vi "数据查询_仪器数据.vi"() -> ()   [LabVIEW 2016]
uses:
  <vilib>/Utility/miscctls.llb/LVRowAndColumnUnsignedTypeDef.ctl
  <vilib>/Utility/miscctls.llb/LVPointTypeDef.ctl
  <userlib>/_OpenG.lib/array/array.llb/Sort 2D Array (String)__ogtk.vi
  <userlib>/_OpenG.lib/array/array.llb/Sort 1D Array (I32)__ogtk.vi
panel:
  in  "下拉列表":string(xcontrol)
  in  "导出":bool
  out "数据筛选_分钟小时":string(combo)="实时数据"
  out "数据筛选_工作类型":string(combo)="全部数据"
  in  "查询":bool
  in  "结束日期":string="2050/01/01"
  in  "起始日期":string="2010/01/01"
  in  "数据表":T1
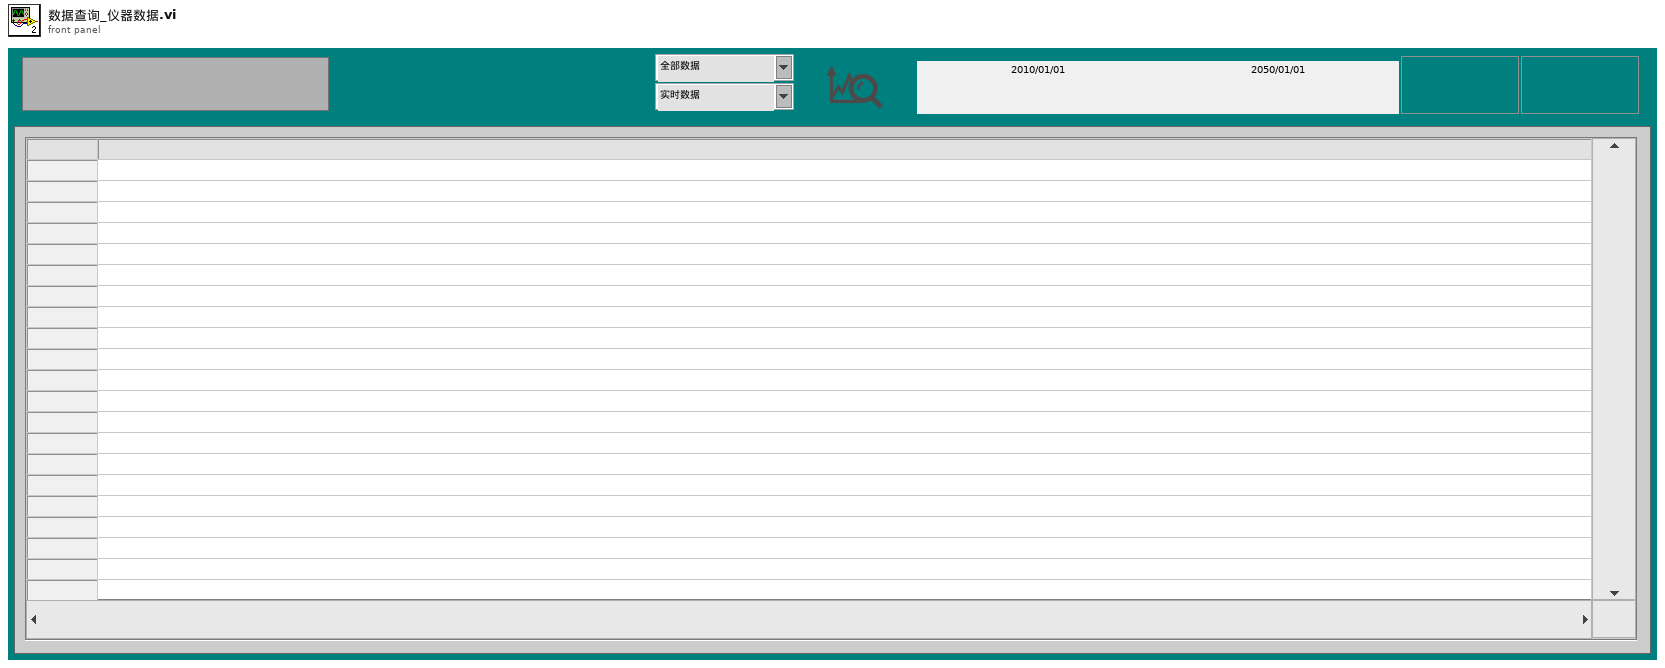
[diagram p1: front panel]
types:
  T1 = typedef "数据查询大列表框.ctl" = i32
  T2 = enum16{"Not Moving", "Mouse Down", "Douse Up", "Moving"}
  T3 = typedef "LVRowAndColumnUnsignedTypeDef.ctl" = cluster{"Row":u32, "Column":u32}
  T4 = typedef "LVPointTypeDef.ctl" = cluster{"Horizontal":i16, "Vertical":i16}
  T5 = cluster{"时间标识":timestamp, "设备":string, "日志信息":string, "流程参数":string}
  T6 = typedef "LVPoint32TypeDef.ctl" = cluster{"Horizontal":i32, "Vertical":i32}
  T7 = typedef "LVRowAndColumnTypeDef.ctl" = cluster{"Row":i32, "Column":i32}
  T8 = enum8{"Enabled", "Disabled", "Disabled and Grayed Out"}
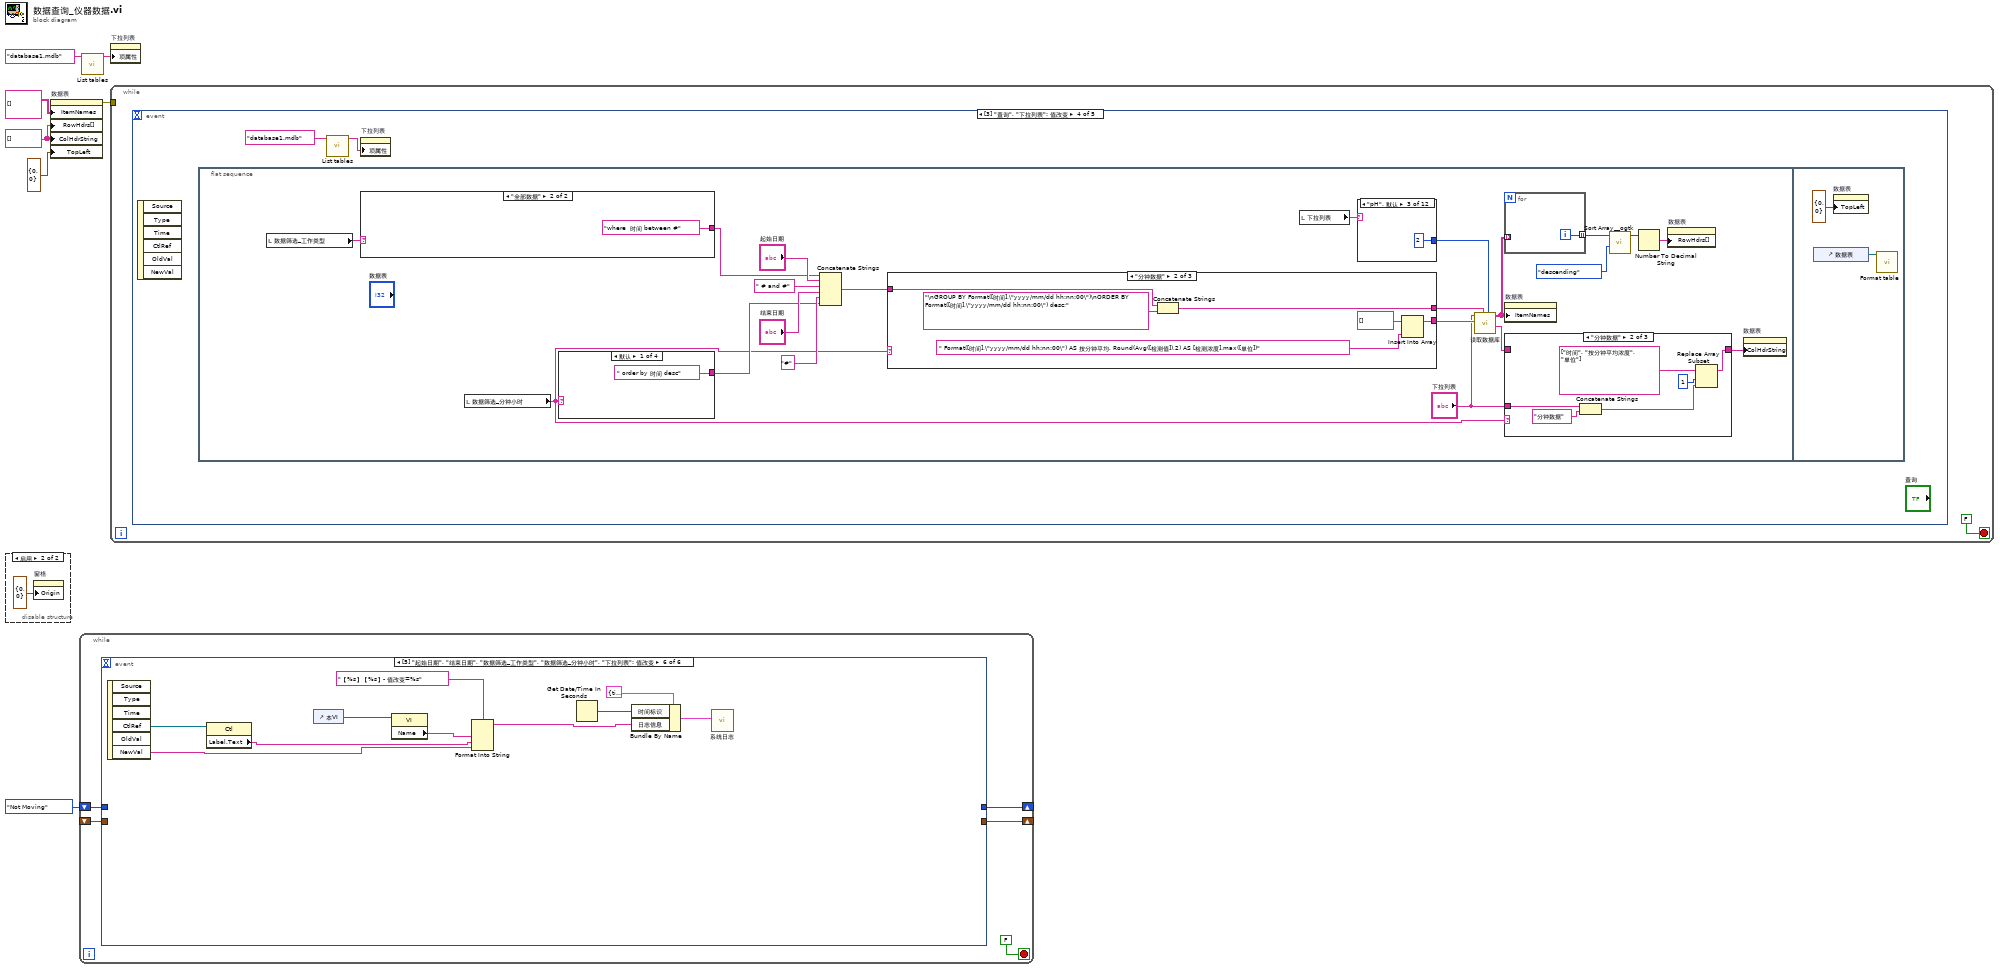
[diagram p0: block diagram]
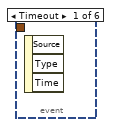
[diagram p2: hidden frame]
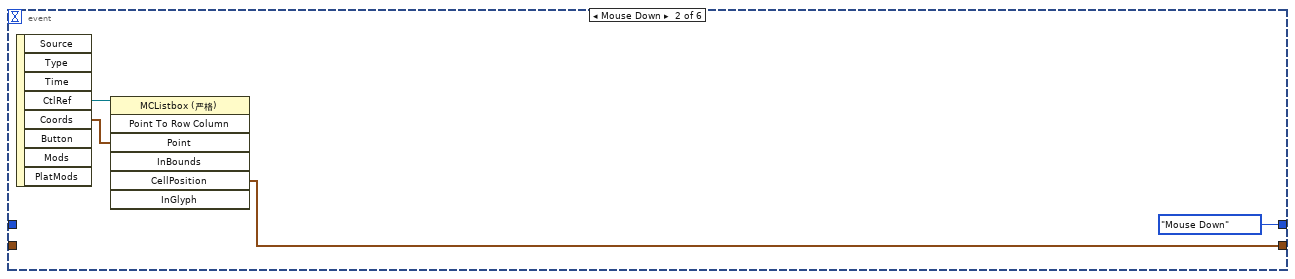
[diagram p3: hidden frame]
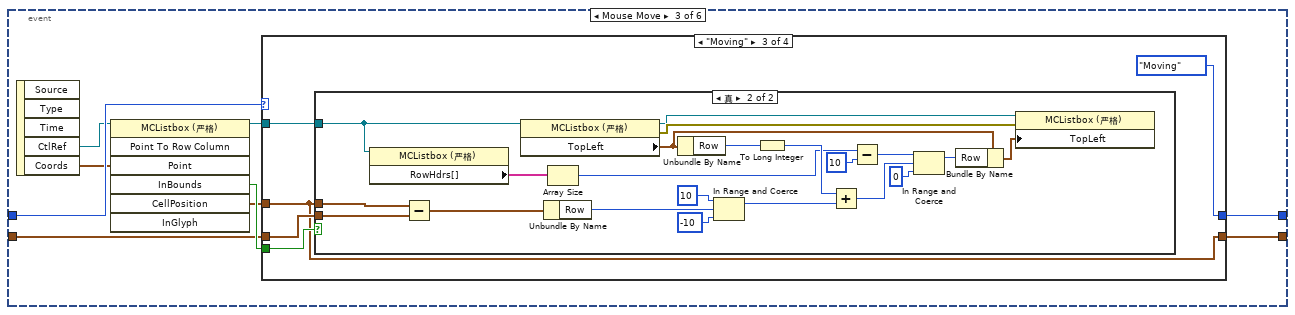
[diagram p4: hidden frame]
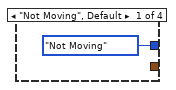
[diagram p5: hidden frame]
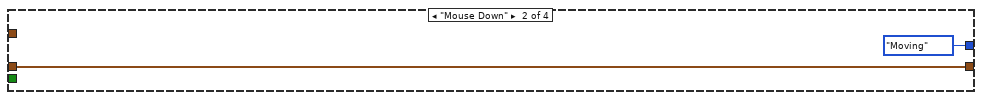
[diagram p6: hidden frame]
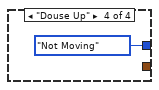
[diagram p8: hidden frame]
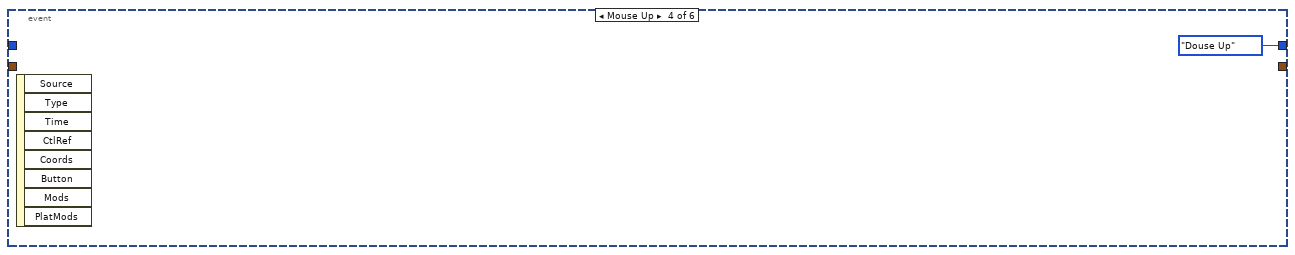
[diagram p9: hidden frame]
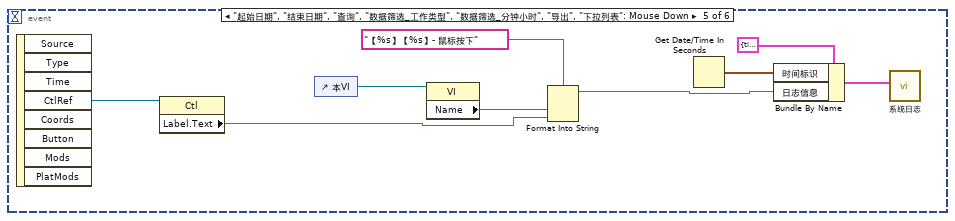
[diagram p10: hidden frame]
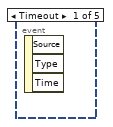
[diagram p11: hidden frame]
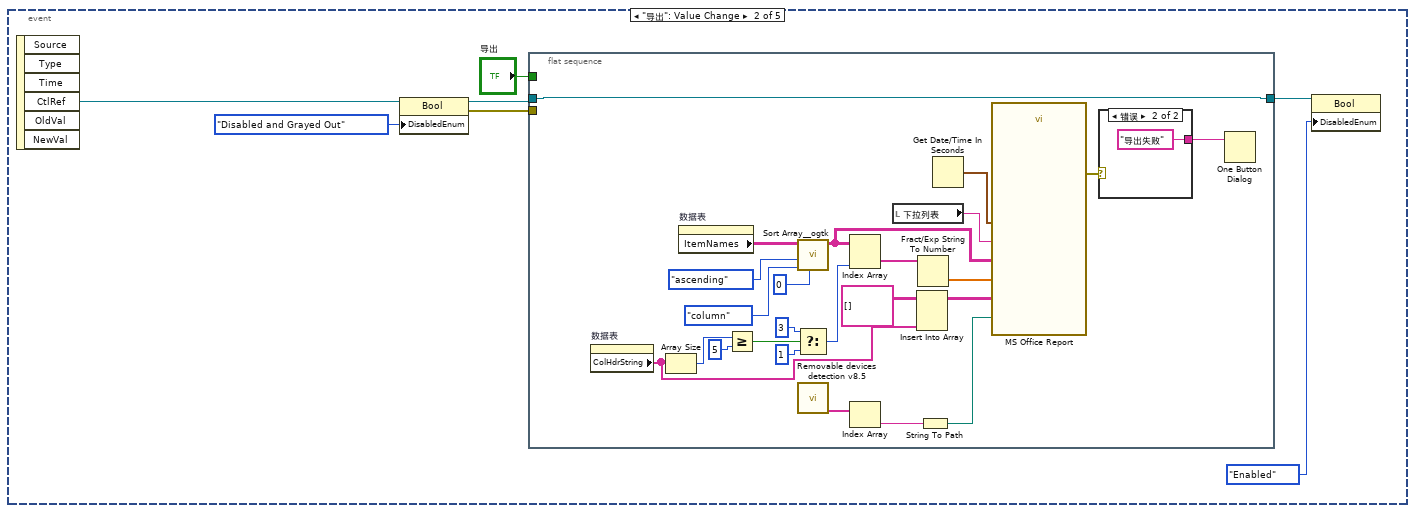
[diagram p12: hidden frame]
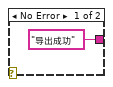
[diagram p13: hidden frame]
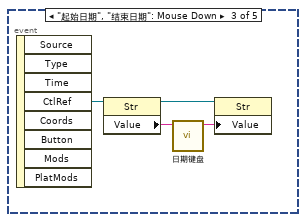
[diagram p14: hidden frame]
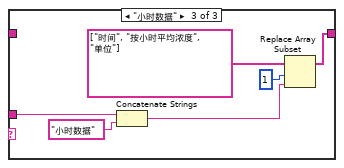
[diagram p16: hidden frame]
diagram:
  w3 = string[] [] ("行首字符串[]")
  n1 = disable-structure shown="启用" {
    frame Disabled {
    }
    frame Enabled {
      n2 = property on="窗格" class="Pane"("Origin"=T4 {"Horizontal"=0, "Vertical"=0} ("原点")) -> ()  [unwired: 2 in, 2 out]
    }
  }
  n3 = property on="数据表" class="MCListbox (严格)"("ItemNames"=string[][] [] ("项名"), "RowHdrs[]"=w3, "ColHdrString"=w3, "TopLeft"=T3 {"Row"=0, "Column"=0} ("左上可见单元格")) -> (error out=w5:errorcluster)  [unwired: 2 in, 1 out]
  n4 = while {
    shift-right: [w11] -> _
    shift-left: T2."Not Moving" -> [w12]
    shift-right: [w10] -> _
    shift-left: _ -> [w9]
    stop <- FALSE stop-if-true
    n5 = event shown="[5] \"起始日期\", \"结束日期\", \"数据筛选_工作类型\", \"数据筛选_分钟小时\", \"下拉列表\": 值改变" {
      selector: _ -> [_ _ _ _ _ _]
      dyn-events: _ -> [_ _ _ _ _ _]
      timeout: _ -> [_ _ _ _ _ _]
      tunnel: w12 -> [_ _ w26 _ _ _]
      tunnel: [_ enum16{"Not Moving", "Mouse Down", "Douse Up"}."Mouse Down" w24 T2."Douse Up" _ _] -> w11
      tunnel: [_ w14 w25 _ _ _] -> w10
      tunnel: w9 -> [_ _ w19 _ _ _]
      event Timeout {
        n6 = event-data() -> ()  [unwired: 1 in, 3 out]
      }
      event Mouse Down {
        n7 = event-data() -> ("CtlRef"=w16:refnum<vi>, "Coords"=w15:T6)  [unwired: 1 in, 6 out]
        n8 = invoke class="MCListbox (严格)" method="Point To Row Column"(reference=w16, "Point"=w15) -> ("CellPosition"=w14:T7)  [unwired: 5 in, 6 out]
      }
      event Mouse Move {
        n9 = event-data() -> ("CtlRef"=w23:refnum<vi>, "Coords"=w22:T6)  [unwired: 1 in, 3 out]
        n10 = invoke class="MCListbox (严格)" method="Point To Row Column"(reference=w23, "Point"=w22) -> (reference out=w18:refnum<vi>, "InBounds"=w21:bool, "CellPosition"=w20:T7)  [unwired: 5 in, 4 out]
        n11 = case shown="\"Moving\"" w26 {
          tunnel: [_ w28 w31 _] -> w25
          tunnel: w19 -> [_ w28 w32 _]
          tunnel: [T2."Not Moving" T2."Moving" T2."Moving" T2."Not Moving"] -> w24
          tunnel: w21 -> [_ _ w33 _]
          tunnel: w20 -> [_ _ w31 _]
          tunnel: w18 -> [_ _ w30 _]
          frame "Not Moving", Default {
          }
          frame "Mouse Down" {
          }
          frame "Moving" {
            n12 = case shown="真" w33 {
              tunnel: w31 -> [_ w55]
              tunnel: w32 -> [_ w54]
              tunnel: w30 -> [_ w35]
              frame False {
              }
              frame True {
                n13 = property on="属性节点" class="MCListbox (严格)"(reference=w35) -> ("RowHdrs[]"=w46:string[])  [unwired: 1 in, 2 out]
                n14 = Subtract(x=w55, y=w54) -> (x-y=w50:T7)
                n15 = property on="属性节点" class="MCListbox (严格)"(reference=w35) -> (reference out=w36:refnum<vi>, error out=w53:errorcluster, "TopLeft"=w52:T3)  [unwired: 1 in]
                n16 = Unbundle By Name(w50) -> ("Row"=w43:i32)
                n17 = Array Size(array=w46) -> (size(s)=w38:i32)
                n18 = Unbundle By Name(w52) -> ("Row"=w45:u32)
                n19 = In Range and Coerce(upper limit=10 ("上限"), x=w43, lower limit=-10 ("下限")) -> (coerced(x)=w40:i32)  [unwired: 1 out]
                n20 = To Long Integer(number=w45) -> (32bit integer=w44:i32)
                n21 = Add(x=w44, y=w40) -> (x+y=w49:i32)
                n22 = Subtract(x=w38, y=10) -> (x-y=w39:i32)
                n23 = In Range and Coerce(upper limit=w39, x=w49, lower limit=0 ("下限")) -> (coerced(x)=w47:i32)  [unwired: 1 out]
                n24 = Bundle By Name(cluster=w52, "Row"=w47) -> (w51:T3)
                n25 = property on="属性节点" class="MCListbox (严格)"(reference=w36, error in=w53, "TopLeft"=w51) -> ()  [unwired: 2 out]
              }
            }
          }
          frame "Douse Up" {
          }
        }
      }
      event Mouse Up {
        n26 = event-data() -> ()  [unwired: 1 in, 8 out]
      }
      event "起始日期", "结束日期", "查询", "数据筛选_工作类型", "数据筛选_分钟小时", "导出", "下拉列表": Mouse Down {
        n27 = event-data() -> ("CtlRef"=w63:refnum<vi>)  [unwired: 1 in, 7 out]
        n28 = property class="Ctl"(reference=w63) -> ("Label.Text"=w62:string)  [unwired: 1 in, 2 out]
        n29 = control-ref of="本VI"() -> (w66:refnum<vi>)
        n30 = property class="VI"(reference=w66) -> ("Name"=w65:string)  [unwired: 1 in, 2 out]
        n31 = Format Into String(format string="【%s】【%s】- 鼠标按下" ("格式字符串"), w65, w62) -> (resulting string=w59:string)  [unwired: 2 in, 1 out]
        n32 = Get Date/Time In Seconds() -> (seconds since 1Jan1904=w58:timestamp)
        n33 = Bundle By Name(cluster=T5 {"时间标识"=timestamp(0 s since 1904-01-01), "设备"="系统", "日志信息"="", "流程参数"=""} ("data in"), "时间标识"=w58, "日志信息"=w59) -> (w60:T5)
        n34 = call "系统日志.vi"("data in"=w60) -> ()  [unwired: 11 in]
      }
      event "起始日期", "结束日期", "数据筛选_工作类型", "数据筛选_分钟小时", "下拉列表": Value Change {
        n35 = event-data() -> ("CtlRef"=w68:refnum<vi>, "NewVal"=w67:string)  [unwired: 1 in, 4 out]
        n36 = property class="Ctl"(reference=w68) -> ("Label.Text"=w73:string)  [unwired: 1 in, 2 out]
        n37 = control-ref of="本VI"() -> (w76:refnum<vi>)
        n38 = property class="VI"(reference=w76) -> ("Name"=w75:string)  [unwired: 1 in, 2 out]
        n39 = Format Into String(format string="【%s】【%s】- 值改变=%s" ("格式字符串"), w75, w73, w67) -> (resulting string=w70:string)  [unwired: 2 in, 1 out]
        n40 = Get Date/Time In Seconds() -> (seconds since 1Jan1904=w69:timestamp)
        n41 = Bundle By Name(cluster=T5 {"时间标识"=timestamp(0 s since 1904-01-01), "设备"="系统", "日志信息"="", "流程参数"=""} ("data in"), "时间标识"=w69, "日志信息"=w70) -> (w71:T5)
        n42 = call "系统日志.vi"("data in"=w71) -> ()  [unwired: 11 in]
      }
    }
  }
  n43 = call "List tables.vi"("database"="database1.mdb") -> ("tables"=w6:string[])  [unwired: 9 in, 1 out]
  n44 = while {
    tunnel: w5 -> [_]
    stop <- FALSE stop-if-true
    n45 = event shown="[3] \"查询\", \"下拉列表\": 值改变" {
      selector: _ -> [_ _ _ _ _]
      dyn-events: _ -> [_ _ _ _ _]
      timeout: _ -> [_ _ _ _ _]
      event Timeout {
        n46 = event-data() -> ()  [unwired: 1 in, 3 out]
      }
      event "导出": Value Change {
        n47 = event-data() -> ("CtlRef"=w78:refnum<vi>)  [unwired: 1 in, 5 out]
        n48 = property class="Bool"(reference=w78, "DisabledEnum"=T8."Disabled and Grayed Out" ("禁用")) -> (reference out=w82:refnum<vi>, error out=w83:errorcluster)  [unwired: 1 in]
        n49 = flat-sequence {
          tunnel: w83 -> [_]
          tunnel: [w100] -> w81
          tunnel: w82 -> [w100]
          tunnel: "导出" -> [_]
          frame #0 {
            n50 = property on="数据表" class="MCListbox (严格)"() -> ("ColHdrString"=w87:string[])  [unwired: 2 in, 2 out]
            n51 = Array Size(array=w87) -> (size(s)=w94:i32)
            n52 = property on="数据表" class="MCListbox (严格)"() -> ("ItemNames"=w85:string[][])  [unwired: 2 in, 2 out]
            n53 = Greater Or Equal?(x=w94, y=5) -> (x >= y?=w92:bool)
            n54 = call-poly <userlib>:"Sort Array__ogtk.vi"("Column/Row to Sort By"=u32 0, "Sort By in"=enum16{"row", "column"}."column", "Order"=enum16{"ascending", "descending"}."ascending", "Array in"=w85) -> ("Sorted Array out"=w107:string[][])  [unwired: 4 in, 3 out]
            n55 = Select(t=3 ("禁用的索引 (列)"), s=w92, f=1) -> (s? t:f=w90:i32)
            n56 = call "Removable devices detection v8.5.vi"() -> ("Removable"=w97:string[])  [unwired: 4 out]
            n57 = Index Array(array=w107, index (col)=w90) -> (element=w103:string[])  [unwired: 1 in]
            n58 = Index Array(array=w97) -> (element=w96:string)  [unwired: 1 in]
            n59 = local read "下拉列表"() -> (w101:string)
            n60 = Insert Into Array(array=string[][] [], new element=w87) -> (w86:string[][])  [unwired: 2 in]
            n61 = Fract/Exp String To Number(string=w103) -> (number=w102:dbl[])  [unwired: 3 in, 1 out]
            n62 = String To Path(string=w96) -> (path=w95:path)
            n63 = Get Date/Time In Seconds() -> (seconds since 1Jan1904=w108:timestamp)
            n64 = call "MS Office Report"("Path to Save Report"=w95, "导出日期"=w108, "监测参数"=w101, "数据输入"=w107, "图表输入"=w102, "字段定义"=w86) -> ("error out"=w99:errorcluster)  [unwired: 20 in, 1 out]
            n65 = case shown="错误" w99 {
              tunnel: ["导出成功" ("消息") "导出失败" ("消息")] -> w98
              frame No Error {
              }
              frame Error {
              }
            }
            n66 = One Button Dialog(message=w98) -> ()  [unwired: 1 in, 1 out]
          }
        }
        n67 = property class="Bool"(reference=w81, "DisabledEnum"=T8."Enabled" ("禁用")) -> ()  [unwired: 1 in, 2 out]
      }
      event "起始日期", "结束日期": Mouse Down {
        n68 = event-data() -> ("CtlRef"=w114:refnum<vi>)  [unwired: 1 in, 7 out]
        n69 = property class="Str"(reference=w114) -> (reference out=w112:refnum<vi>, "Value"=w113:string)  [unwired: 1 in, 1 out]
        n70 = call "日期键盘.vi"("原值"=w113) -> ("x+y"=w111:string)  [unwired: 10 in]
        n71 = property class="Str"(reference=w112, "Value"=w111) -> ()  [unwired: 1 in, 2 out]
      }
      event "查询", "下拉列表": Value Change {
        n72 = event-data() -> ()  [unwired: 1 in, 6 out]
        n73 = flat-sequence {
          frame #0 {
            n74 = local read "数据筛选_工作类型"() -> (w129:string)
            n75 = case shown="\"全部数据\"" w129 {
              selector: w129 -> [w167 _]
              tunnel: [w165 "where  时间 between #" ("condition")] -> w128
              frame Default {
                n76 = Format Into String(format string="where 测量模式 ='%s' and 时间 between #" ("condition"), w167) -> (resulting string=w165:string)  [unwired: 2 in, 1 out]
              }
              frame "全部数据" {
              }
            }
            n77 = local read "数据筛选_分钟小时"() -> (w123:string)
            n78 = case shown="默认" w123 {
              tunnel: [" order by 时间 desc" ("字符串") _ _ _] -> w127
              frame Default {
              }
              frame "分钟数据" {
              }
              frame "小时数据" {
              }
              frame "真" {
              }
            }
            n79 = Concatenate Strings(w128, "起始日期", " # and #" ("condition"), "结束日期", "#" ("condition"), w127) -> (w126:string)
            n80 = case shown="\"分钟数据\"" w123 {
              tunnel: [_ w157 w159] -> w124
              tunnel: w126 -> [w152 w155 w161]
              tunnel: [w152 w154 w160] -> w125
              frame Default {
              }
              frame "分钟数据" {
                n81 = Concatenate Strings(w155, "\nGROUP BY Format([时间],\"yyyy/mm/dd hh:nn:00\")\nORDER BY Format([时间],\"yyyy/mm/dd hh:nn:00\") desc;" ("字符串")) -> (w154:string)
                n82 = Insert Into Array(array=string[] [] ("显示项"), new element=" Format([时间],\"yyyy/mm/dd hh:nn:00\") AS 按分钟平均, Round(Avg([检测值]),2) AS [检测浓度],max([单位])" ("新元素/子数组")) -> (w157:string[])  [unwired: 1 in]
              }
              frame "小时数据" {
                n83 = Concatenate Strings(w161, "\nGROUP BY Format([时间],\"yyyy/mm/dd hh:00:00\")\nORDER BY Format([时间],\"yyyy/mm/dd hh:00:00\") desc;" ("字符串")) -> (w160:string)
                n84 = Insert Into Array(array=string[] [] ("显示项"), new element=" Format([时间],\"yyyy/mm/dd hh:00:00\") AS 按分钟平均, Round(Avg([检测值]),2) AS [检测浓度],max([单位])" ("新元素/子数组")) -> (w159:string[])  [unwired: 1 in]
              }
            }
            n85 = local read "下拉列表"() -> (w131:string)
            n86 = case shown="\"pH\", 默认" w131 {
              tunnel: [i16 3 ("精度(6)") i16 1 ("精度(6)") i16 2 ("精度(6)") i16 2 ("精度(6)") i16 2 ("精度(6)") i16 2 ("精度(6)") i16 2 ("精度(6)") i16 2 ("精度(6)") i16 3 ("精度(6)") i16 2 ("精度(6)") i16 2 ("精度(6)") i16 2 ("精度(6)")] -> w130
              frame "氨氮" {
              }
              frame "水温" {
              }
              frame "pH", Default {
              }
              frame "溶解氧" {
              }
              frame "电导率" {
              }
              frame "浊度" {
              }
              frame "藻密度" {
              }
              frame "叶绿素a" {
              }
              frame "总磷" {
              }
              frame "总氮" {
              }
              frame "CodCr" {
              }
              frame "CodMn" {
              }
            }
            n87 = call "读取数据库.vi"("精度(6)"=w130, "condition"=w125, "显示项"=w124, "组合框"="下拉列表") -> ("columns"=w122:string[], "表格"=w117:string[][])  [unwired: 4 in, 2 out]
            n88 = for {
              tunnel: w117 -> [_] mode=indexing
              tunnel: [w181] -> w133 mode=indexing
              i -> [w181]
            }
            n89 = property on="数据表" class="MCListbox (严格)"("ItemNames"=w117) -> ()  [unwired: 2 in, 2 out]
            n90 = case shown="\"分钟数据\"" w123 {
              tunnel: w122 -> [w138 _ _]
              tunnel: [w138 w142 w146] -> w121
              tunnel: "下拉列表" -> [_ w141 w147]
              frame Default {
              }
              frame "分钟数据" {
                n91 = Concatenate Strings(w141, "分钟数据" ("字符串")) -> (w139:string)
                n92 = Replace Array Subset(array=string[] ["时间", "按分钟平均浓度", "单位"] ("columns"), new element=w139, index=1 ("索引")) -> (w142:string[])
              }
              frame "小时数据" {
                n93 = Concatenate Strings(w147, "小时数据" ("字符串")) -> (w148:string)
                n94 = Replace Array Subset(array=string[] ["时间", "按小时平均浓度", "单位"] ("columns"), new element=w148, index=1 ("索引")) -> (w146:string[])
              }
            }
            n95 = call-poly <userlib>:"Sort Array__ogtk.vi"("Order"=enum16{"ascending", "descending"}."descending", "Array in"=w133) -> ("Sorted Array out"=w118:i32[])  [unwired: 8 in, 1 out]
            n96 = Number To Decimal String(number=w118) -> (decimal integer string=w132:string[])  [unwired: 1 in]
            n97 = property on="数据表" class="MCListbox (严格)"("RowHdrs[]"=w132) -> ()  [unwired: 2 in, 2 out]
            n98 = property on="数据表" class="MCListbox (严格)"("ColHdrString"=w121) -> ()  [unwired: 2 in, 2 out]
          }
          frame #1 {
            n99 = control-ref of="数据表"() -> (w182:refnum<vi>)
            n100 = property on="数据表" class="MCListbox (严格)"("TopLeft"=T3 {"Row"=0, "Column"=0} ("索引值")) -> ()  [unwired: 2 in, 2 out]
            n101 = call "Format table.vi"("Table输入"=w182) -> ()  [unwired: 11 in]
          }
        }
        n102 = call "List tables.vi"("database"="database1.mdb") -> ("tables"=w115:string[])  [unwired: 9 in, 1 out]
        n103 = property on="下拉列表" class="下拉列表 (严格)"("项属性"=w115) -> ()  [unwired: 2 in, 2 out]
      }
      event "数据筛选_工作类型", "数据筛选_分钟小时": Mouse Down {
        n104 = event-data() -> ()  [unwired: 1 in, 8 out]
        n105 = call "数据查询筛选.vi"() -> ("分钟小时"=w184:string, "工作类型"=w185:string)  [unwired: 10 in]
        "数据筛选_工作类型" <- w185
        "数据筛选_分钟小时" <- w184
        n106 = property on="数据筛选_工作类型" class="CmbBox"("Val(Sgnl)"=w185) -> ()  [unwired: 2 in, 2 out]
        n107 = property on="数据筛选_分钟小时" class="CmbBox"("Val(Sgnl)"=w184) -> ()  [unwired: 2 in, 2 out]
      }
    }
  }
  n108 = property on="下拉列表" class="下拉列表 (严格)"("项属性"=w6) -> ()  [unwired: 2 in, 2 out]
